vi "eMIC PF.vi"(11 "eMIC 1":T1) -> (3 "output cluster":T1)   [LabVIEW 2018, in "Application.lvlib"]
uses:
  Application.lvlib
  eMIC response.ctl
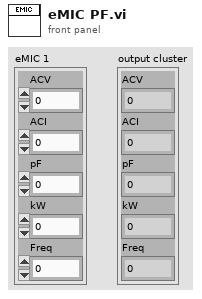
[diagram p1: front panel]
types:
  T1 = typedef "Application.lvlib/eMIC response.ctl" = cluster{"ACV":dbl, "ACI":dbl, "pF":dbl, "kW":dbl, "Freq":dbl}
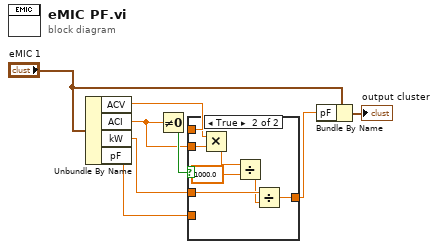
[diagram p0: block diagram]
diagram:
  n1 = Unbundle By Name("eMIC 1") -> ("ACV"=w2:dbl, "ACI"=w5:dbl, "kW"=w3:dbl, "pF"=w7:dbl)
  n2 = Not Equal To 0?(x=w5) -> (x != 0?=w6:bool)
  n3 = case shown="True" w6 {
    tunnel: w2 -> [_ w16]
    tunnel: w3 -> [_ w13]
    tunnel: [w9 w11] -> w4
    tunnel: w5 -> [_ w10]
    tunnel: w7 -> [w9 _]
    frame False {
    }
    frame True {
      n4 = Multiply(x=w16, y=w10) -> (x*y=w15:dbl)
      n5 = Divide(x=w15, y=1000.0) -> (x/y=w12:dbl)
      n6 = Divide(x=w13, y=w12) -> (x/y=w11:dbl)
    }
  }
  n7 = Bundle By Name(cluster="eMIC 1", "pF"=w4) -> (→"output cluster":T1)
